vi "for_v0_v3.vi"() -> ()   [LabVIEW 2010]
panel:
  out "Numeric":dbl
  in  "stop":bool
  out "Array":bool[](array[boolean])=[FALSE, TRUE, FALSE, FALSE, TRUE, FALSE, TRUE, TRUE]
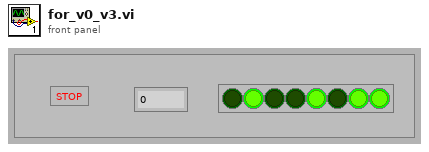
[diagram p1: front panel]
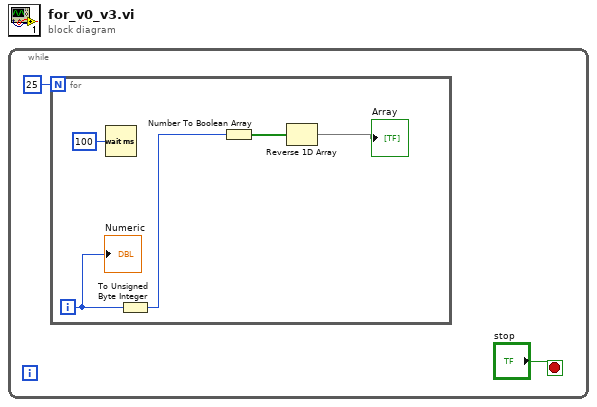
[diagram p0: block diagram]
diagram:
  n1 = while {
    stop <- "stop" stop-if-true
    n2 = for {
      N: 25 -> [_]
      i -> [w3]
      n3 = Wait (ms)(milliseconds to wait=u32 100) -> ()  [unwired: 1 out]
      n4 = To Unsigned Byte Integer(number=w3) -> (unsigned 8bit integer=w4:u8)
      n5 = Number To Boolean Array(number=w4) -> (Boolean array=w7:bool[])
      n6 = Reverse 1D Array(array=w7) -> (reversed array=→"Array":bool[])
      "Numeric" <- w3
    }
  }
